vi "Set all panes to their origin.vi"(8 "error in (no error)":errorcluster, 11 "Top level VI ref":refnum<vi>) -> (0 "error out":errorcluster)   [LabVIEW 2017]
uses:
  <vilib>/Utility/miscctls.llb/LVPointTypeDef.ctl
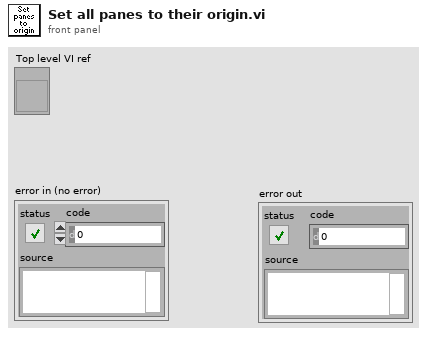
[diagram p1: front panel]
types:
  T1 = typedef "LVPointTypeDef.ctl" = cluster{"Horizontal":i16, "Vertical":i16}
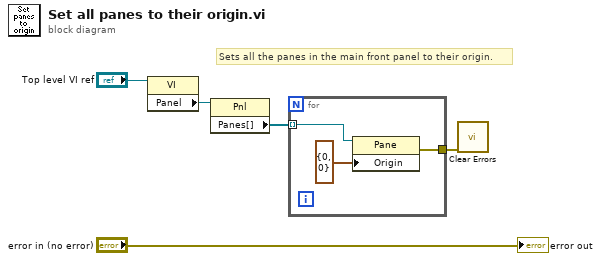
[diagram p0: block diagram]
diagram:
  # "Sets all the panes in the main front panel to their origin."
  n1 = property class="VI"(reference="Top level VI ref") -> ("Panel"=w3:refnum<vi>)  [unwired: 1 in, 2 out]
  n2 = property class="Pnl"(reference=w3) -> ("Panes[]"=w2:refnum<vi>[])  [unwired: 1 in, 2 out]
  n3 = for {
    tunnel: [w7] -> w5
    tunnel: w2 -> [w6] mode=indexing
    n4 = property class="Pane"(reference=w6, "Origin"=T1 {"Horizontal"=0, "Vertical"=0}) -> (error out=w7:errorcluster)  [unwired: 1 in, 1 out]
  }
  n5 = call <vilib>:"Clear Errors.vi"("error in (no error)"=w5) -> ()  [unwired: 5 in, 2 out]
  "error out" <- "error in (no error)"
